vi "Result_Test.vi"(8 "error in (no error)":errorcluster caption="entrée d'erreur (pas d'erreur)", 11 "Delay en entrée":refnum<class "Generate_Install_Code.lvclass">) -> (0 "error out":errorcluster caption="sortie d'erreur", 3 "Delay en sortie":refnum<class "Generate_Install_Code.lvclass">)   [LabVIEW 2020, in "Library Test.lvlib" / "Generate_Install_Code.lvclass"]
uses:
  Generate_Install_Code.lvclass
  C:/Users/ngarcin/OneDrive - Altyor/Standard TB/Suite TB45/Class/Test/Test (Default)/Test (Default).lvclass
  Commun VI/TypeDef/Variable Printable.ctl
  Test_Without_Instr/Test_Without_Inst.lvclass
  Commun VI/Library Commun.lvlib
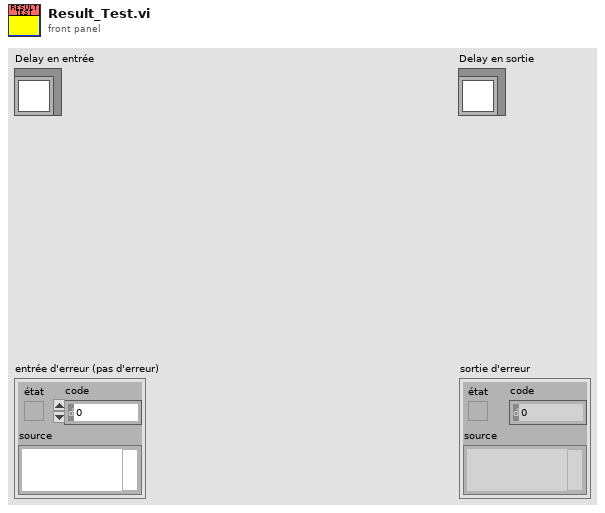
[diagram p1: front panel]
types:
  T1 = typedef "Variable Printable.ctl" = string
  T2 = enum16{"Get Variable", "Get All Variables", "Set Variable", "Delete Variable", "Delete All Variable"}
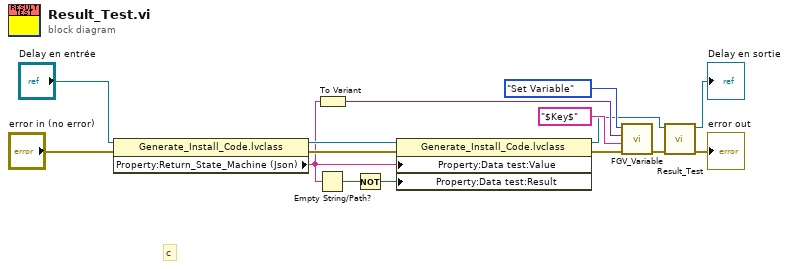
[diagram p0: block diagram]
diagram:
  # "c"
  n1 = property class="Generate_Install_Code.lvclass"(reference="Delay en entrée", error in="error in (no error)") -> (reference out=w10:refnum<class "Generate_Install_Code.lvclass">, error out=w9:errorcluster, "Property:Return_State_Machine (Json)"=w1:string)
  n2 = Empty String/Path?(string/path=w1) -> (empty?=w3:bool)
  n3 = To Variant(anything=w1) -> (Variant=w13:variant)
  n4 = Not(x=w3) -> (.not. x?=w2:bool)
  n5 = property class="Generate_Install_Code.lvclass"(reference=w10, error in=w9, "Property:Data test:Value"=w1, "Property:Data test:Result"=w2) -> (reference out=w4:refnum<class "Generate_Install_Code.lvclass">, error out=w6:errorcluster)
  n6 = call "FGV_Variable.vi"("error in (no error)"=w6, "Variable"=T1 "$Key$" ("Variable Printable"), "Data In"=w13, "Function"=T2."Set Variable") -> ("error out"=w7:errorcluster)  [unwired: 5 in, 2 out]
  n7 = call-parent "Result_Test.vi"("error in (no error)"=w7, "Test_Without_Inst en entrée"=w4) -> ("error out"=→"error out":errorcluster, "Test_Without_Inst en sortie"=→"Delay en sortie":refnum<class "Generate_Install_Code.lvclass">)  [unwired: 8 in]
